vi "Read Messenger.vi"(11 "API in":refnum<class "API.lvclass">) -> (3 "Messenger":refnum<user-event>)   [LabVIEW 2024, in "API.lvclass"]
uses:
  API.lvclass
  API.lvclass/API.ctl
  Message.ctl
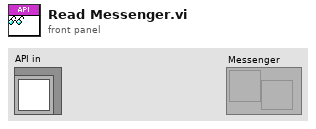
[diagram p1: front panel]
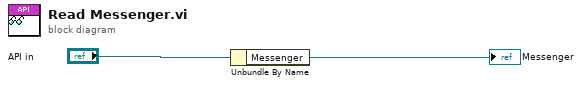
[diagram p0: block diagram]
diagram:
  n1 = Unbundle By Name("API in") -> ("Messenger"=→"Messenger":refnum<user-event>)
